vi "SubVI_Path2Fig_001.vi"(1 "length (rest)":i32=3, 2 "Path":path) -> (0 "FIG":string)   [LabVIEW 2018]
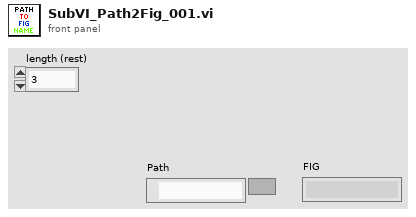
[diagram p1: front panel]
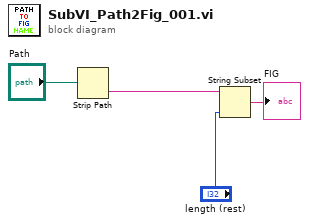
[diagram p0: block diagram]
diagram:
  n1 = Strip Path(path="Path") -> (name=w2:string)  [unwired: 1 out]
  n2 = String Subset(string=w2, length (rest)="length (rest)") -> (substring=→"FIG":string)  [unwired: 1 in]
